vi "SendToDash.vi"   [LabVIEW 2018]
uses:
  Subsystems/Drive/MotionProfile/AutoOptions.ctl
  Subsystems/Drive/MotionProfile/StartingPosition.ctl
  Subsystems/Drive/MotionProfile/Path_Decider.ctl
  <userlib>/836-Library/System/TDMS_V2/Support/TDMS_DevRef.ctl
  <userlib>/836-Library/System/TDMS_V2/Support/Logging_Settings.ctl
  <userlib>/836-Library/System/TDMS_V2/Support/Group_FIFO_Config.ctl
  <userlib>/836-Library/System/TDMS_V2/Support/Channel_FIFO_Config.ctl
  <vilib>/Rock Robotics/Network Tables/NT Read Variant.vi
  <vilib>/Rock Robotics/Network Tables/NT Write Boolean.vi
  <vilib>/Rock Robotics/Network Tables/NT Write String.vi
  <vilib>/Rock Robotics/Network Tables/NT Write Number.vi
  <vilib>/Rock Robotics/WPI/ThirdParty/Phoenix-LabVIEW/Motor Controller/Get/CTRE_Phoenix_MotorController_GetSelectedSensorData.vi
types:
  T1 = typedef "WPI_DigitalInputDevRef.ctl" = cluster{"DevStatus":errorcluster, "DIO Channel":T2}
  T2 = typedef "FPGA_DIOChannel.ctl" = enum8{"DIO 0", "DIO 1", "DIO 2", "DIO 3", "DIO 4", "DIO 5", "DIO 6", "DIO 7", "DIO 8", "DIO 9", "DIO MXP 0", "DIO MXP 1", "DIO MXP 2", "DIO MXP 3", "DIO MXP 4", "DIO MXP 5", "DIO MXP 6", "DIO MXP 7", "DIO MXP 8", "DIO MXP 9", "DIO MXP 10", "DIO MXP 11", "DIO MXP 12", "DIO MXP 13", "DIO MXP 14", "DIO MXP 15", "SPI Port CS1", "SPI Port CS2", "SPI Port CS3", "SPI Port MISO", "SPI Port MOSI", "Invalid"}
  T3 = cluster{"proportional gain (Kc)":dbl, "integral time (Ti, min)":dbl, "derivative time (Td, min)":dbl}
  T4 = typedef "WPI_MotorControlDeviceRef.ctl" = cluster{"DeviceStatus":errorcluster, "Type":T5, "PWM":cluster{"PWM Channel":T6, "DeadBand":T7}, "CAN":cluster{"Device Number":u8, "SetOutput VI Ref":variant, "GetOutput VI Ref":variant, "Enable VI Ref":variant, "Disable VI Ref":variant, "Data":variant}, "Invert":bool, "DIO PWM":cluster{"PWM \"Enable\" Channel":T6, "DIOChannel":T2, "PWM Rate":dbl}}
  T5 = typedef "WPI_MotorControlType.ctl" = enum16{"PWM", "CAN", "DIO PWM"}
  T6 = typedef "FPGA_DIOPWMChannel.ctl" = enum8{"PWM 0", "PWM 1", "PWM 2", "PWM 3", "PWM 4", "PWM 5", "PWM 6", "PWM 7", "PWM 8", "PWM 9", "PWM MXP 0", "PWM MXP 1", "PWM MXP 2", "PWM MXP 3", "PWM MXP 4", "PWM MXP 5", "PWM MXP 6", "PWM MXP 7", "PWM MXP 8", "PWM MXP 9", "Invalid"}
  T7 = typedef "WPI_PWMDeadband.ctl" = cluster{"Name":string, "maxPositivePwm":i32, "minPositivePwm":i32, "centerPwm":i32, "maxNegativePwm":i32, "minNegativePwm":i32, "angularRange":u16}
  T8 = typedef "AutoOptions.ctl" = cluster{"Starting Position":T9, "First Score Pos":T10, "Second Score Pos":T10}
  T9 = typedef "StartingPosition.ctl" = enum16{"Left L1 ", "Middle L1", "Right L1", "Left L2", "Right L2", "Don't Move"}
  T10 = typedef "Path_Decider.ctl" = enum16{"1", "2", "3", "4", "5", "6", "7", "8", "Left_Rocket_Front", "Left_Rocket_Rear", "Right_Rocket_Front", "Right_Rocket_Rear"}
  T11 = typedef "NetComm_MatchType.ctl" = enum32{"None", "Practice", "Qualification", "Elimination"}
  T12 = typedef "WPI_AnalogChannelDevRef.ctl" = cluster{"DevStatus":errorcluster, "Analog Channel":T13}
  T13 = typedef "FPGA_AIChannel.ctl" = enum8{"AI 0", "AI 1", "AI 2", "AI 3", "AI MXP 0", "AI MXP 1", "AI MXP 2", "AI MXP 3", "Invalid"}
  T14 = typedef "TDMS_DevRef.ctl" = cluster{"Name":string, "File Ref":refnum<k34>, "Start Time":timestamp, "Logging Settings":T15, "Group FIFO Config":T16[], "Data To Write":refnum<data-value>, "semaphore":T18, "Ref Time Reset":refnum<k4>}
  T15 = typedef "Logging_Settings.ctl" = cluster{"Data Grab Period":dbl, "File Write Period":dbl, "Max Stored Size":dbl, "Burst Size":dbl}
  T16 = typedef "Group_FIFO_Config.ctl" = cluster{"Group":string, "Channels":T17[], "Channel Names":string[]}
  T17 = typedef "Channel_FIFO_Config.ctl" = cluster{"Channel":string, "FIFO":refnum<k33>}
  T18 = typedef "Semaphore RefNum" = refnum<k1>
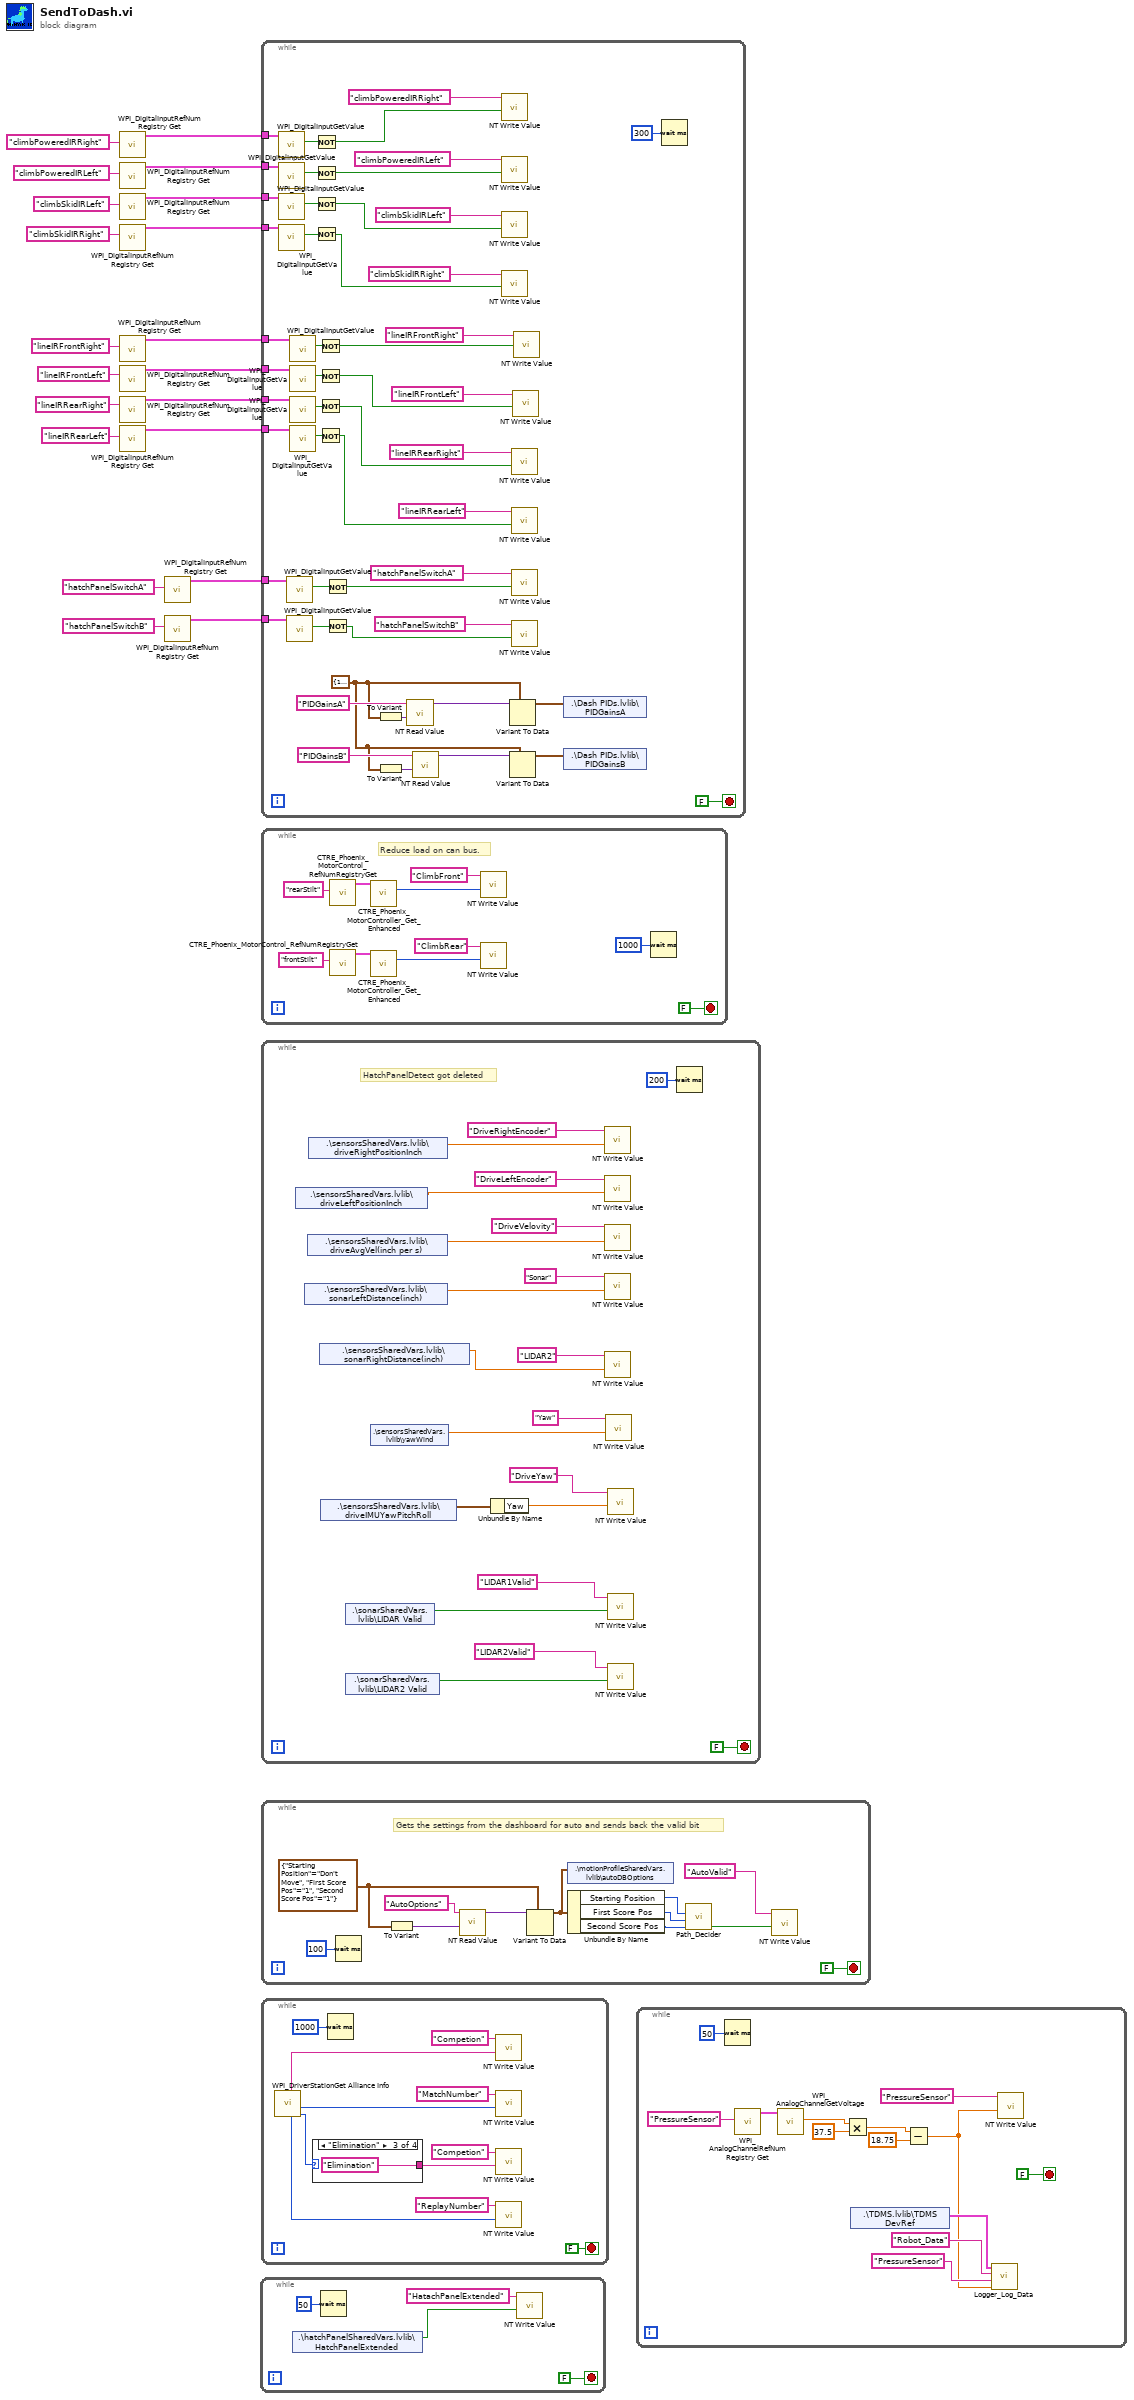
[diagram p0: block diagram]
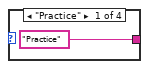
[diagram p2: hidden frame]
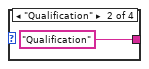
[diagram p3: hidden frame]
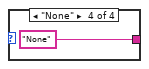
[diagram p4: hidden frame]
diagram:
  n1 = call <vilib>:"WPI_DigitalInputRefNum Registry Get.vi"("refnum name"="climbPoweredIRRight") -> ("DigitalInputDevRef"=w16:T1)  [unwired: 9 in, 1 out]
  n2 = call <vilib>:"WPI_DigitalInputRefNum Registry Get.vi"("refnum name"="climbPoweredIRLeft") -> ("DigitalInputDevRef"=w15:T1)  [unwired: 9 in, 1 out]
  n3 = call <vilib>:"WPI_DigitalInputRefNum Registry Get.vi"("refnum name"="climbSkidIRLeft") -> ("DigitalInputDevRef"=w14:T1)  [unwired: 9 in, 1 out]
  n4 = call <vilib>:"WPI_DigitalInputRefNum Registry Get.vi"("refnum name"="climbSkidIRRight") -> ("DigitalInputDevRef"=w13:T1)  [unwired: 9 in, 1 out]
  n5 = call <vilib>:"WPI_DigitalInputRefNum Registry Get.vi"("refnum name"="lineIRFrontRight") -> ("DigitalInputDevRef"=w8:T1)  [unwired: 9 in, 1 out]
  n6 = call <vilib>:"WPI_DigitalInputRefNum Registry Get.vi"("refnum name"="lineIRFrontLeft") -> ("DigitalInputDevRef"=w5:T1)  [unwired: 9 in, 1 out]
  n7 = call <vilib>:"WPI_DigitalInputRefNum Registry Get.vi"("refnum name"="lineIRRearRight") -> ("DigitalInputDevRef"=w6:T1)  [unwired: 9 in, 1 out]
  n8 = call <vilib>:"WPI_DigitalInputRefNum Registry Get.vi"("refnum name"="lineIRRearLeft") -> ("DigitalInputDevRef"=w7:T1)  [unwired: 9 in, 1 out]
  n9 = call <vilib>:"WPI_DigitalInputRefNum Registry Get.vi"("refnum name"="hatchPanelSwitchA") -> ("DigitalInputDevRef"=w2:T1)  [unwired: 9 in, 1 out]
  n10 = call <vilib>:"WPI_DigitalInputRefNum Registry Get.vi"("refnum name"="hatchPanelSwitchB") -> ("DigitalInputDevRef"=w1:T1)  [unwired: 9 in, 1 out]
  n11 = while {
    stop <- FALSE stop-if-true
    n12 = shared-variable ".\\hatchPanelSharedVars.lvlib\\HatchPanelExtended"() -> (w22:bool)  [unwired: 1 in, 1 out]
    n13 = Wait (ms)(milliseconds to wait=i64 50 ("Period")) -> ()  [unwired: 1 out]
    n14 = call-poly <vilib>:"NT Write Value.vi"("Boolean"=w22, "Name"="HatachPanelExtended") -> ()  [unwired: 9 in, 1 out]
  }
  n15 = while {
    tunnel: w16 -> [w67]
    tunnel: w15 -> [w66]
    tunnel: w14 -> [w65]
    tunnel: w13 -> [w64]
    tunnel: w8 -> [w55]
    tunnel: w7 -> [w54]
    tunnel: w6 -> [w53]
    tunnel: w5 -> [w52]
    tunnel: w2 -> [w41]
    tunnel: w1 -> [w40]
    stop <- FALSE stop-if-true
    w27 = T3 {"proportional gain (Kc)"=1.0, "integral time (Ti, min)"=0.01, "derivative time (Td, min)"=0.0} ("PID gains")
    n16 = call <vilib>:"WPI_DigitalInputGetValue.vi"("DigitalInputDevRef"=w67) -> ("Value"=w68:bool)  [unwired: 8 in, 2 out]
    n17 = call <vilib>:"WPI_DigitalInputGetValue.vi"("DigitalInputDevRef"=w66) -> ("Value"=w69:bool)  [unwired: 8 in, 2 out]
    n18 = call <vilib>:"WPI_DigitalInputGetValue.vi"("DigitalInputDevRef"=w65) -> ("Value"=w70:bool)  [unwired: 8 in, 2 out]
    n19 = call <vilib>:"WPI_DigitalInputGetValue.vi"("DigitalInputDevRef"=w64) -> ("Value"=w71:bool)  [unwired: 8 in, 2 out]
    n20 = call <vilib>:"WPI_DigitalInputGetValue.vi"("DigitalInputDevRef"=w41) -> ("Value"=w43:bool)  [unwired: 8 in, 2 out]
    n21 = call <vilib>:"WPI_DigitalInputGetValue.vi"("DigitalInputDevRef"=w40) -> ("Value"=w42:bool)  [unwired: 8 in, 2 out]
    n22 = call <vilib>:"WPI_DigitalInputGetValue.vi"("DigitalInputDevRef"=w55) -> ("Value"=w59:bool)  [unwired: 8 in, 2 out]
    n23 = call <vilib>:"WPI_DigitalInputGetValue.vi"("DigitalInputDevRef"=w52) -> ("Value"=w58:bool)  [unwired: 8 in, 2 out]
    n24 = call <vilib>:"WPI_DigitalInputGetValue.vi"("DigitalInputDevRef"=w53) -> ("Value"=w57:bool)  [unwired: 8 in, 2 out]
    n25 = call <vilib>:"WPI_DigitalInputGetValue.vi"("DigitalInputDevRef"=w54) -> ("Value"=w56:bool)  [unwired: 8 in, 2 out]
    n26 = Not(x=w68) -> (.not. x?=w63:bool)
    n27 = Not(x=w69) -> (.not. x?=w62:bool)
    n28 = Not(x=w70) -> (.not. x?=w61:bool)
    n29 = Not(x=w71) -> (.not. x?=w60:bool)
    n30 = Not(x=w59) -> (.not. x?=w47:bool)
    n31 = Not(x=w58) -> (.not. x?=w46:bool)
    n32 = Not(x=w57) -> (.not. x?=w45:bool)
    n33 = Not(x=w56) -> (.not. x?=w44:bool)
    n34 = Not(x=w43) -> (.not. x?=w37:bool)
    n35 = Not(x=w42) -> (.not. x?=w36:bool)
    n36 = To Variant(anything=w27) -> (Variant=w29:variant)
    n37 = To Variant(anything=w27) -> (Variant=w28:variant)
    n38 = call-poly <vilib>:"NT Read Value.vi"("Default Value"=w29, "Name"="PIDGainsA") -> ("Variant"=w33:variant)  [unwired: 8 in, 1 out]
    n39 = call-poly <vilib>:"NT Read Value.vi"("Default Value"=w28, "Name"="PIDGainsB") -> ("Variant"=w32:variant)  [unwired: 8 in, 1 out]
    n40 = call-poly <vilib>:"NT Write Value.vi"("Boolean"=w63, "Name"="climbPoweredIRRight") -> ()  [unwired: 9 in, 1 out]
    n41 = call-poly <vilib>:"NT Write Value.vi"("Boolean"=w62, "Name"="climbPoweredIRLeft") -> ()  [unwired: 9 in, 1 out]
    n42 = call-poly <vilib>:"NT Write Value.vi"("Boolean"=w61, "Name"="climbSkidIRLeft") -> ()  [unwired: 9 in, 1 out]
    n43 = call-poly <vilib>:"NT Write Value.vi"("Boolean"=w60, "Name"="climbSkidIRRight") -> ()  [unwired: 9 in, 1 out]
    n44 = Variant To Data(type=w27, Variant=w33) -> (data=w31:T3)  [unwired: 1 in, 1 out]
    n45 = Variant To Data(type=w27, Variant=w32) -> (data=w30:T3)  [unwired: 1 in, 1 out]
    n46 = call-poly <vilib>:"NT Write Value.vi"("Boolean"=w45, "Name"="lineIRRearRight") -> ()  [unwired: 9 in, 1 out]
    n47 = call-poly <vilib>:"NT Write Value.vi"("Boolean"=w44, "Name"="lineIRRearLeft") -> ()  [unwired: 9 in, 1 out]
    n48 = call-poly <vilib>:"NT Write Value.vi"("Boolean"=w37, "Name"="hatchPanelSwitchA") -> ()  [unwired: 9 in, 1 out]
    n49 = call-poly <vilib>:"NT Write Value.vi"("Boolean"=w36, "Name"="hatchPanelSwitchB") -> ()  [unwired: 9 in, 1 out]
    n50 = call-poly <vilib>:"NT Write Value.vi"("Boolean"=w46, "Name"="lineIRFrontLeft") -> ()  [unwired: 9 in, 1 out]
    n51 = call-poly <vilib>:"NT Write Value.vi"("Boolean"=w47, "Name"="lineIRFrontRight") -> ()  [unwired: 9 in, 1 out]
    n52 = shared-variable ".\\Dash PIDs.lvlib\\PIDGainsA"(w31) -> ()  [unwired: 1 in, 1 out]
    n53 = shared-variable ".\\Dash PIDs.lvlib\\PIDGainsB"(w30) -> ()  [unwired: 1 in, 1 out]
    n54 = Wait (ms)(milliseconds to wait=i64 300 ("Period")) -> ()  [unwired: 1 out]
  }
  n55 = while {
    stop <- FALSE stop-if-true
    # "Reduce load on can bus."
    n56 = call <vilib>:"CTRE_Phoenix_MotorControl_RefNumRegistryGet.vi"("refnum name"="rearStilt") -> ("PhoenixMotorControlDevRef"=w83:T4)  [unwired: 9 in, 1 out]
    n57 = call <vilib>:"CTRE_Phoenix_MotorControl_RefNumRegistryGet.vi"("refnum name"="frontStilt") -> ("PhoenixMotorControlDevRef"=w82:T4)  [unwired: 9 in, 1 out]
    n58 = call-poly <vilib>:"CTRE_Phoenix_MotorController_Get_Enhanced.vi"("PhoenixMotorControlDevRef"=w83) -> ("Position (Raw Sensor Units)"=w79:i32)  [unwired: 11 in, 3 out]
    n59 = call-poly <vilib>:"CTRE_Phoenix_MotorController_Get_Enhanced.vi"("PhoenixMotorControlDevRef"=w82) -> ("Position (Raw Sensor Units)"=w78:i32)  [unwired: 11 in, 3 out]
    n60 = call-poly <vilib>:"NT Write Value.vi"("Numeric"=w79, "Name"="ClimbFront") -> ()  [unwired: 9 in, 1 out]
    n61 = call-poly <vilib>:"NT Write Value.vi"("Numeric"=w78, "Name"="ClimbRear") -> ()  [unwired: 9 in, 1 out]
    n62 = Wait (ms)(milliseconds to wait=i64 1000 ("Period")) -> ()  [unwired: 1 out]
  }
  n63 = while {
    stop <- FALSE stop-if-true
    # "HatchPanelDetect got deleted"
    n64 = shared-variable ".\\sensorsSharedVars.lvlib\\driveLeftPositionInch"() -> (w96:dbl)  [unwired: 1 in, 1 out]
    n65 = shared-variable ".\\sensorsSharedVars.lvlib\\sonarLeftDistance(inch)"() -> (w98:dbl)  [unwired: 1 in, 1 out]
    n66 = shared-variable ".\\sensorsSharedVars.lvlib\\driveAvgVel(inch per s)"() -> (w106:dbl)  [unwired: 1 in, 1 out]
    n67 = shared-variable ".\\sensorsSharedVars.lvlib\\driveRightPositionInch"() -> (w97:dbl)  [unwired: 1 in, 1 out]
    n68 = shared-variable ".\\sensorsSharedVars.lvlib\\sonarRightDistance(inch)"() -> (w92:dbl)  [unwired: 1 in, 1 out]
    n69 = shared-variable ".\\sensorsSharedVars.lvlib\\driveIMUYawPitchRoll"() -> (w95:cluster{"Yaw":dbl, "Pitch":dbl, "Roll":dbl})  [unwired: 1 in, 1 out]
    n70 = shared-variable ".\\sonarSharedVars.lvlib\\LIDAR Valid"() -> (w90:bool)  [unwired: 1 in, 1 out]
    n71 = shared-variable ".\\sonarSharedVars.lvlib\\LIDAR2 Valid"() -> (w91:bool)  [unwired: 1 in, 1 out]
    n72 = shared-variable ".\\sensorsSharedVars.lvlib\\yawWind"() -> (w99:dbl)  [unwired: 1 in, 1 out]
    n73 = Unbundle By Name(w95) -> ("Yaw"=w94:dbl)
    n74 = call-poly <vilib>:"NT Write Value.vi"("Numeric"=w97, "Name"="DriveRightEncoder") -> ()  [unwired: 9 in, 1 out]
    n75 = call-poly <vilib>:"NT Write Value.vi"("Numeric"=w96, "Name"="DriveLeftEncoder") -> ()  [unwired: 9 in, 1 out]
    n76 = call-poly <vilib>:"NT Write Value.vi"("Numeric"=w106, "Name"="DriveVelovity") -> ()  [unwired: 9 in, 1 out]
    n77 = call-poly <vilib>:"NT Write Value.vi"("Numeric"=w98, "Name"="Sonar") -> ()  [unwired: 9 in, 1 out]
    n78 = call-poly <vilib>:"NT Write Value.vi"("Numeric"=w92, "Name"="LIDAR2") -> ()  [unwired: 9 in, 1 out]
    n79 = call-poly <vilib>:"NT Write Value.vi"("Numeric"=w99, "Name"="Yaw") -> ()  [unwired: 9 in, 1 out]
    n80 = call-poly <vilib>:"NT Write Value.vi"("Numeric"=w94, "Name"="DriveYaw") -> ()  [unwired: 9 in, 1 out]
    n81 = call-poly <vilib>:"NT Write Value.vi"("Boolean"=w90, "Name"="LIDAR1Valid") -> ()  [unwired: 9 in, 1 out]
    n82 = call-poly <vilib>:"NT Write Value.vi"("Boolean"=w91, "Name"="LIDAR2Valid") -> ()  [unwired: 9 in, 1 out]
    n83 = Wait (ms)(milliseconds to wait=i64 200 ("Period")) -> ()  [unwired: 1 out]
  }
  n84 = while {
    stop <- FALSE stop-if-true
    w115 = T8 {"Starting Position"=enum."Don't Move", "First Score Pos"=enum."1", "Second Score Pos"=enum."1"}
    # "Gets the settings from the dashboard for auto and sends back the valid bit"
    n85 = Wait (ms)(milliseconds to wait=i64 100 ("Period")) -> ()  [unwired: 1 out]
    n86 = To Variant(anything=w115) -> (Variant=w116:variant)
    n87 = call-poly <vilib>:"NT Read Value.vi"("Default Value"=w116, "Name"="AutoOptions") -> ("Variant"=w118:variant)  [unwired: 8 in, 1 out]
    n88 = Variant To Data(type=w115, Variant=w118) -> (data=w114:T8)  [unwired: 1 in, 1 out]
    n89 = shared-variable ".\\motionProfileSharedVars.lvlib\\autoDBOptions"(w114) -> ()  [unwired: 1 in, 1 out]
    n90 = Unbundle By Name(w114) -> ("Starting Position"=w113:T9, "First Score Pos"=w112:T10, "Second Score Pos"=w111:T10)
    n91 = call "Path_Decider.vi"("Second"=w111, "First"=w112, "Starting Position"=w113) -> ("Complete Path Valid?"=w110:bool)  [unwired: 4 in, 3 out]
    n92 = call-poly <vilib>:"NT Write Value.vi"("Boolean"=w110, "Name"="AutoValid") -> ()  [unwired: 9 in, 1 out]
  }
  n93 = while {
    stop <- FALSE stop-if-true
    n94 = call <vilib>:"WPI_DriverStationGet Alliance Info.vi"() -> ("Match Type"=w122:T11, "Match Number"=w124:u16, "Replay Number"=w121:u16, "Event Name"=w128:string)  [unwired: 6 in, 2 out]
    n95 = case shown="\"Elimination\"" w122 {
      tunnel: ["Practice" "Qualification" "Elimination" "None"] -> w123
      frame "Practice" {
      }
      frame "Qualification" {
      }
      frame "Elimination" {
      }
      frame "None" {
      }
    }
    n96 = Wait (ms)(milliseconds to wait=i64 1000 ("Period")) -> ()  [unwired: 1 out]
    n97 = call-poly <vilib>:"NT Write Value.vi"("String"=w128, "Name"="Competion") -> ()  [unwired: 9 in, 1 out]
    n98 = call-poly <vilib>:"NT Write Value.vi"("Numeric"=w124, "Name"="MatchNumber") -> ()  [unwired: 9 in, 1 out]
    n99 = call-poly <vilib>:"NT Write Value.vi"("String"=w123, "Name"="Competion") -> ()  [unwired: 9 in, 1 out]
    n100 = call-poly <vilib>:"NT Write Value.vi"("Numeric"=w121, "Name"="ReplayNumber") -> ()  [unwired: 9 in, 1 out]
  }
  n101 = while {
    stop <- FALSE stop-if-true
    n102 = Wait (ms)(milliseconds to wait=i64 50 ("Period")) -> ()  [unwired: 1 out]
    n103 = call <vilib>:"WPI_AnalogChannelRefNum Registry Get.vi"("refnum name"="PressureSensor") -> ("AIDeviceRef"=w145:T12)  [unwired: 9 in, 1 out]
    n104 = call <vilib>:"WPI_AnalogChannelGetVoltage.vi"("AIDeviceRef"=w145) -> ("Voltage"=w140:dbl)  [unwired: 8 in, 2 out]
    n105 = Multiply(x=w140, y=37.5) -> (x*y=w141:dbl)
    n106 = shared-variable ".\\TDMS.lvlib\\TDMS DevRef"() -> (w137:T14)  [unwired: 1 in, 1 out]
    n107 = Subtract(x=w141, y=18.75) -> (x-y=w134:dbl)
    n108 = call <userlib>:"Logger_Log_Data.vi"("Data"=w134, "Channel"="PressureSensor" ("refnum name"), "Group"="Robot_Data", "TDMS DevRef"=w137) -> ()  [unwired: 7 in, 1 out]
    n109 = call-poly <vilib>:"NT Write Value.vi"("Numeric"=w134, "Name"="PressureSensor" ("refnum name")) -> ()  [unwired: 9 in, 1 out]
  }
